vi "Single_Pulse_Debuger.vi"() -> ()   [LabVIEW 2021]
uses:
  Drivers/Arduino_Pulse_Generator/Configurate/Channel_Pulse_Stream.ctl
  Addons/Prepare_Pulse_Sequence/Pulse_Sequence_Global.vi
panel:
  in  "Unit":string(combo)
  in  "Enum":T1(ring)=enum."initialize"
  in  "Arduino VISA":refnum<visa-resource-name>
  out "pulse seq changed (?)":bool=TRUE
  out "Init outp register 2 (8-13)":bool[](array[boolean])
  out "Init outp register 1 (2-7)":bool[](array[boolean])
  out "Pulse sequence":T2[](array[typedef]) {"channel" min=2 max=13 step=1}
  in  "Run sequence":bool
  in  "Close":bool
  in  "Define pulse sequence":bool
  in  "Define initial states":bool
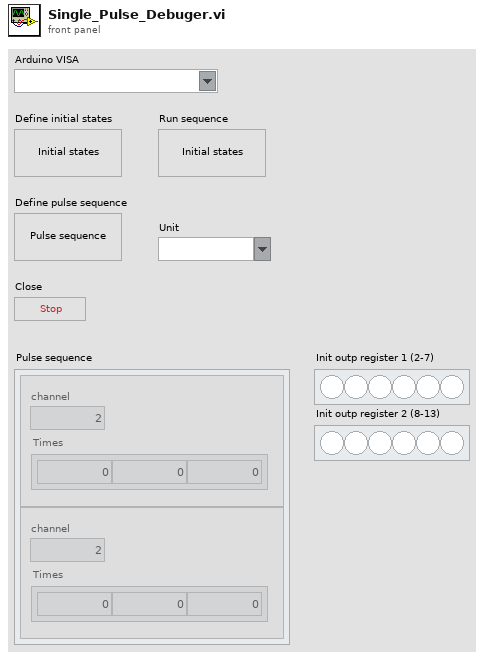
[diagram p1: front panel]
types:
  T1 = enum16{"close", "run", "set pulse", "set initial", "initialize"}
  T2 = typedef "Channel_Pulse_Stream.ctl" = cluster{"Times":dbl[], "channel":u8}
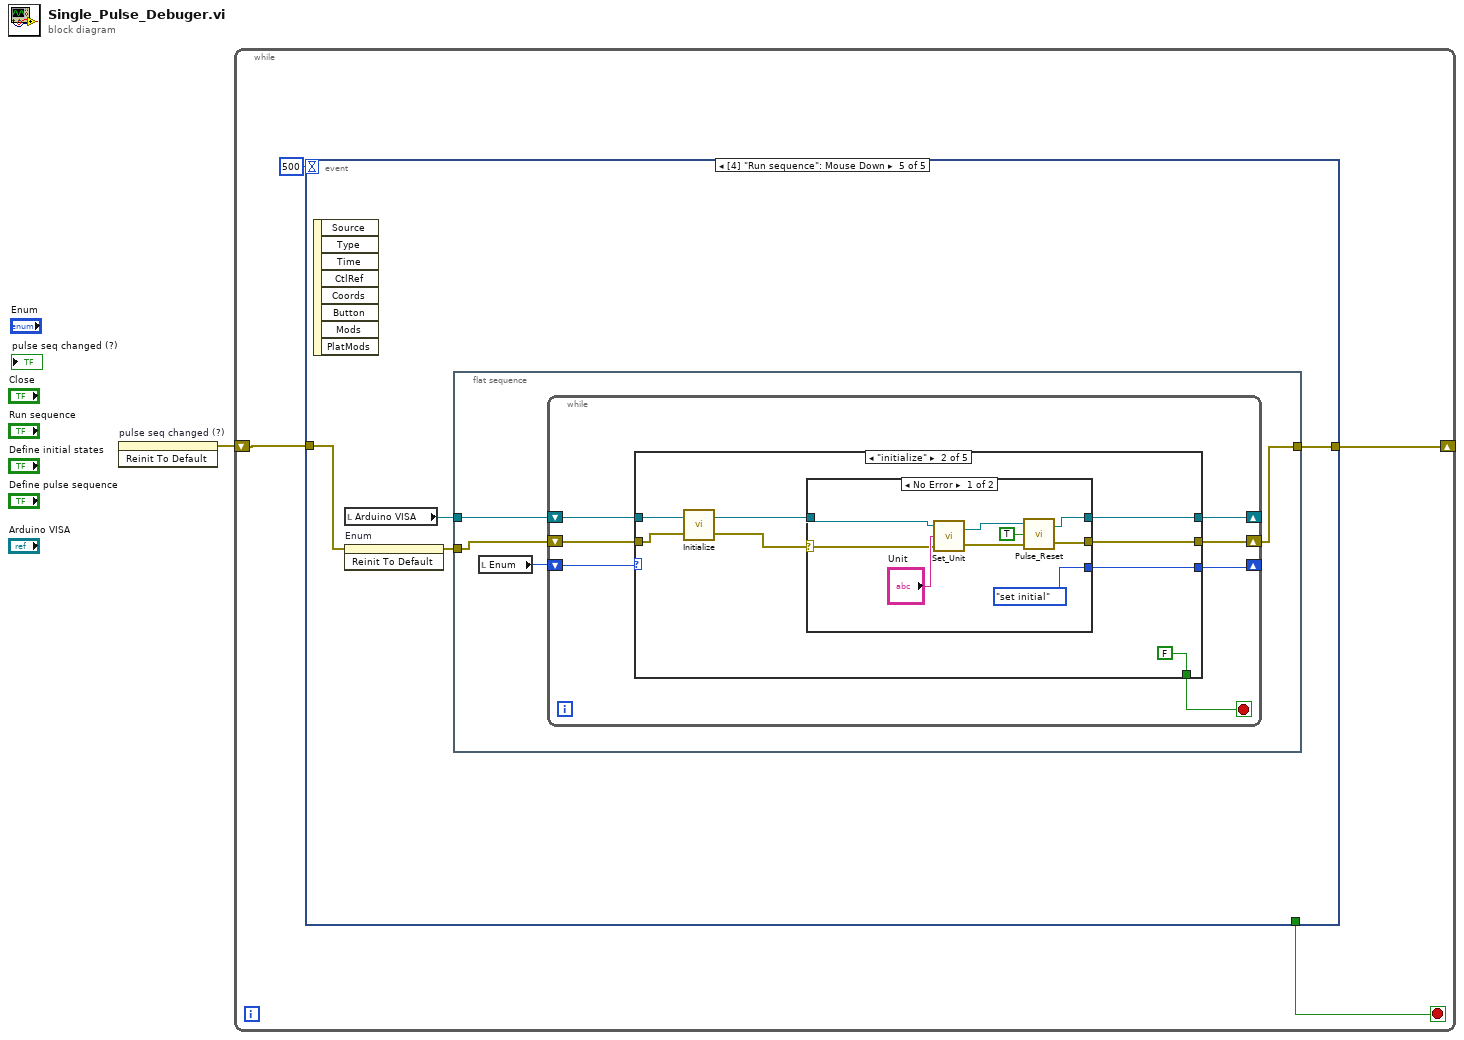
[diagram p0: block diagram]
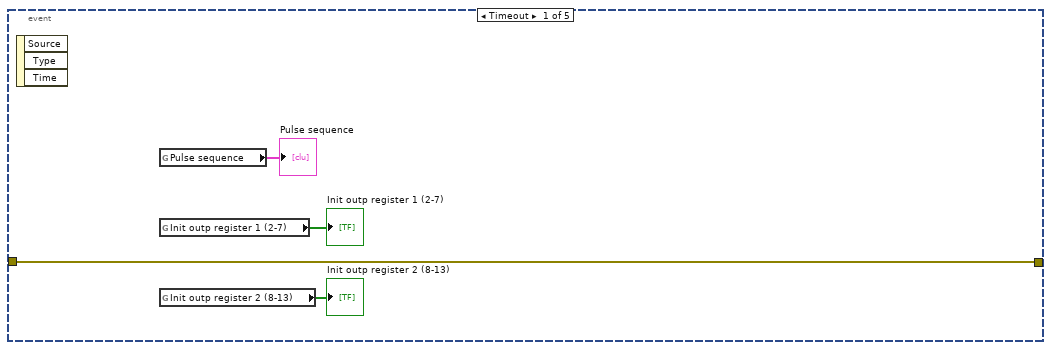
[diagram p2: hidden frame]
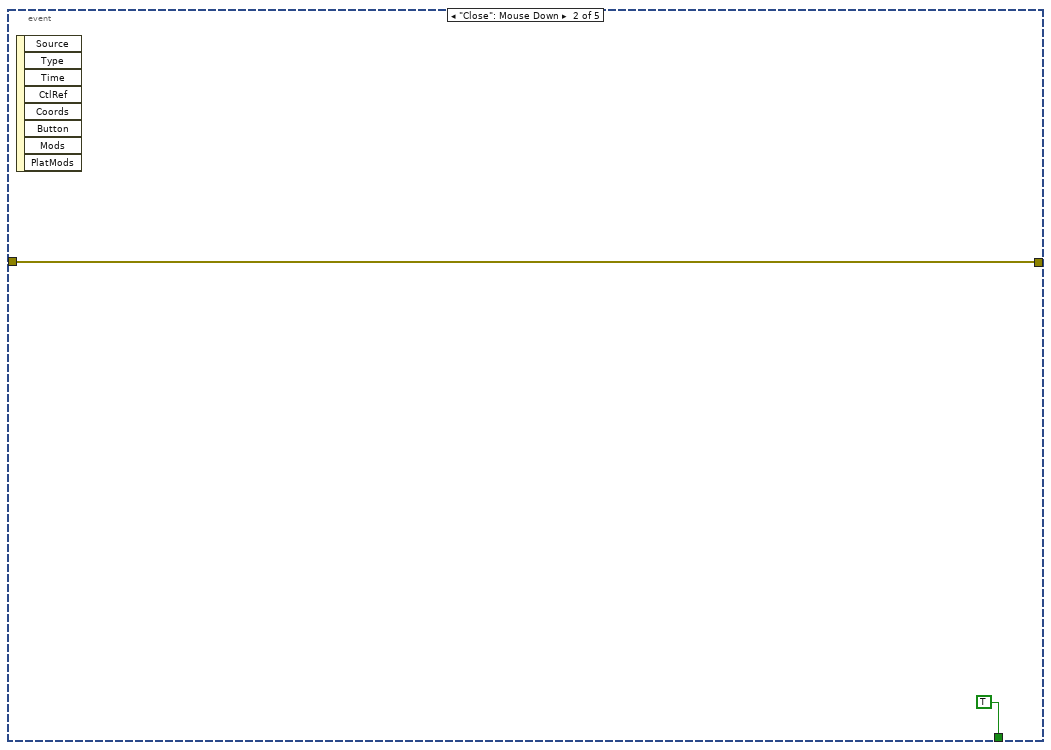
[diagram p3: hidden frame]
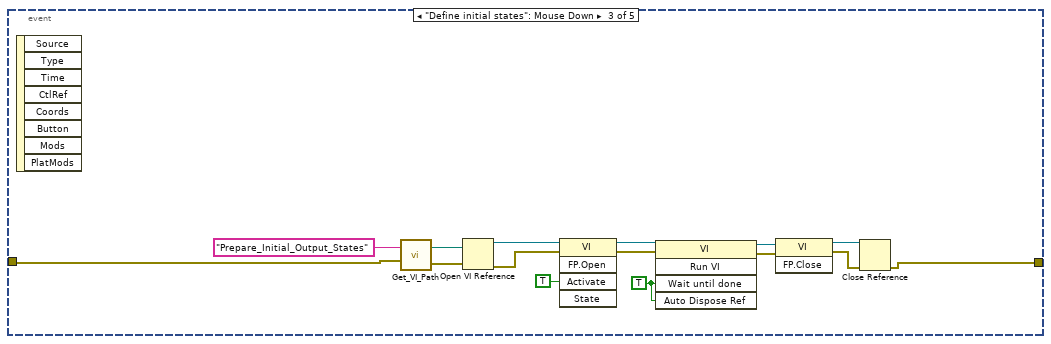
[diagram p4: hidden frame]
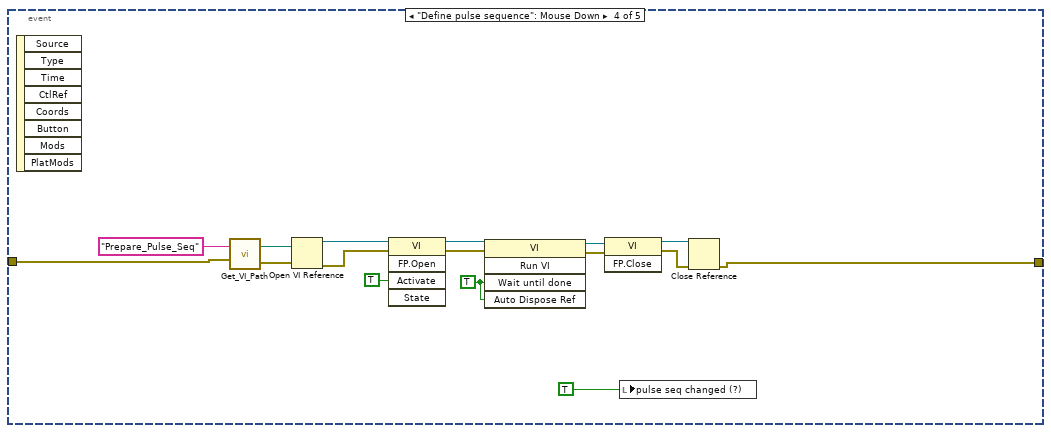
[diagram p5: hidden frame]
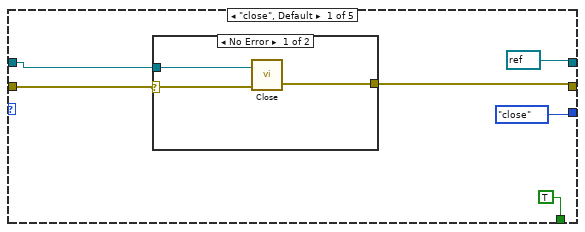
[diagram p6: hidden frame]
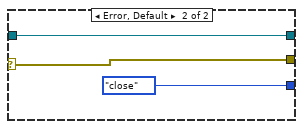
[diagram p8: hidden frame]
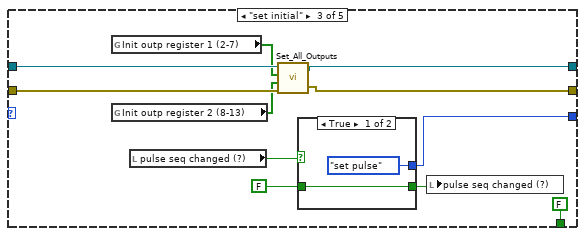
[diagram p9: hidden frame]
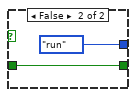
[diagram p10: hidden frame]
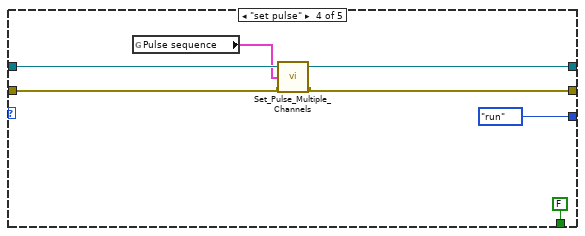
[diagram p11: hidden frame]
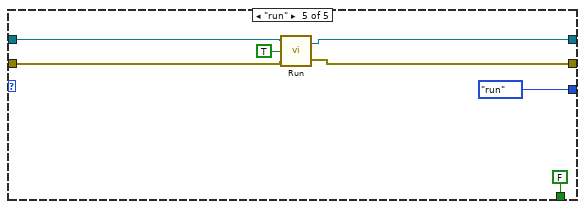
[diagram p12: hidden frame]
diagram:
  n1 = invoke on="pulse seq changed (?)" class="Bool (strict)" method="Reinit To Default"() -> (error out=w1:errorcluster)  [unwired: 3 in, 2 out]
  n2 = while {
    shift-right: [w4] -> _
    shift-left: w1 -> [w5]
    stop <- w2 stop-if-true
    n3 = event shown="[4] \"Run sequence\": Mouse Down" {
      selector: _ -> [_ _ _ _ _]
      dyn-events: _ -> [_ _ _ _ _]
      timeout: 500 -> [_ _ _ _ _]
      tunnel: w5 -> [w6 w10 w13 w29 w44]
      tunnel: [w6 w10 w12 w28 w43] -> w4
      tunnel: [_ TRUE _ _ _] -> w2
      event Timeout {
        n4 = event-data() -> ()  [unwired: 1 in, 3 out]
        n5 = global read "Pulse_Sequence_Global.vi" "Pulse sequence"() -> (→"Pulse sequence":T2[])
        n6 = global read "Pulse_Sequence_Global.vi" "Init outp register 1 (2-7)"() -> (→"Init outp register 1 (2-7)":bool[])
        n7 = global read "Pulse_Sequence_Global.vi" "Init outp register 2 (8-13)"() -> (→"Init outp register 2 (8-13)":bool[])
      }
      event "Close": Mouse Down {
        n8 = event-data() -> ()  [unwired: 1 in, 8 out]
      }
      event "Define initial states": Mouse Down {
        w18 = TRUE ("Wait Until Done")
        n9 = event-data() -> ()  [unwired: 1 in, 8 out]
        n10 = call "Get_VI_Path.vi"("error in"=w13, "VI name (no .vi)"="Prepare_Initial_Output_States") -> ("error out"=w23:errorcluster, "File Path"=w25:path)
        n11 = Open VI Reference(vi path=w25, error in (no error)=w23) -> (vi reference=w24:refnum<vi>, error out=w22:errorcluster)  [unwired: 4 in]
        n12 = invoke class="VI" method="FP.Open"(reference=w24, error in=w22, "Activate"=TRUE ("Activate?")) -> (reference out=w20:refnum<vi>, error out=w19:errorcluster)  [unwired: 2 in, 3 out]
        n13 = invoke class="VI" method="Run VI"(reference=w20, error in=w19, "Wait until done"=w18, "Auto Dispose Ref"=w18) -> (reference out=w17:refnum<vi>, error out=w16:errorcluster)  [unwired: 1 in, 3 out]
        n14 = invoke class="VI" method="FP.Close"(reference=w17, error in=w16) -> (reference out=w15:refnum<vi>, error out=w14:errorcluster)  [unwired: 1 in, 1 out]
        n15 = Close Reference(reference=w15, error in (no error)=w14) -> (error out=w12:errorcluster)
      }
      event "Define pulse sequence": Mouse Down {
        w34 = TRUE ("Wait Until Done")
        n16 = event-data() -> ()  [unwired: 1 in, 8 out]
        n17 = call "Get_VI_Path.vi"("error in"=w29, "VI name (no .vi)"="Prepare_Pulse_Seq") -> ("error out"=w39:errorcluster, "File Path"=w41:path)
        n18 = Open VI Reference(vi path=w41, error in (no error)=w39) -> (vi reference=w40:refnum<vi>, error out=w38:errorcluster)  [unwired: 4 in]
        n19 = invoke class="VI" method="FP.Open"(reference=w40, error in=w38, "Activate"=TRUE ("Activate?")) -> (reference out=w36:refnum<vi>, error out=w35:errorcluster)  [unwired: 2 in, 3 out]
        n20 = invoke class="VI" method="Run VI"(reference=w36, error in=w35, "Wait until done"=w34, "Auto Dispose Ref"=w34) -> (reference out=w33:refnum<vi>, error out=w32:errorcluster)  [unwired: 1 in, 3 out]
        n21 = invoke class="VI" method="FP.Close"(reference=w33, error in=w32) -> (reference out=w31:refnum<vi>, error out=w30:errorcluster)  [unwired: 1 in, 1 out]
        n22 = local write "pulse seq changed (?)"(TRUE ("pulse seq changed (?)")) -> ()
        n23 = Close Reference(reference=w31, error in (no error)=w30) -> (error out=w28:errorcluster)
      }
      event "Run sequence": Mouse Down {
        n24 = event-data() -> ()  [unwired: 1 in, 8 out]
        n25 = local read "Arduino VISA"() -> (w45:refnum<visa-resource-name>)
        n26 = invoke on="Enum" class="Enum (strict)" method="Reinit To Default"(error in=w44) -> (error out=w46:errorcluster)  [unwired: 2 in, 2 out]
        n27 = flat-sequence {
          tunnel: w46 -> [w49]
          tunnel: w45 -> [w50]
          tunnel: [w48] -> w43
          frame #0 {
            n28 = local read "Enum"() -> (w47:T1)
            n29 = while {
              shift-right: [w53] -> _
              shift-left: w47 -> [w51]
              shift-right: [w55] -> _
              shift-left: w50 -> [w57]
              shift-right: [w54] -> w48
              shift-left: w49 -> [w56]
              stop <- w52 stop-if-true
              n30 = case shown="\"initialize\"" w51 {
                tunnel: w57 -> [w63 w75 w97 w105 w115]
                tunnel: w56 -> [w59 w69 w95 w108 w113]
                tunnel: [refnum<visa-resource-name> refnum ("Arduino VISA") w74 w96 w106 w114] -> w55
                tunnel: [w62 w73 w94 w107 w112] -> w54
                tunnel: [T1."close" ("Enum") w72 w98 T1."run" ("Enum") T1."run" ("Enum")] -> w53
                tunnel: [TRUE FALSE FALSE FALSE FALSE] -> w52
                frame "close", Default {
                  n31 = case shown="No Error" w59 {
                    selector: w59 -> [w64 w67]
                    tunnel: w63 -> [w66 _]
                    tunnel: [w65 w67] -> w62
                    frame No Error {
                      n32 = call "Close.vi"("error in"=w64, "VISA arduino in"=w66) -> ("error out"=w65:errorcluster)  [unwired: 1 in]
                    }
                    frame Error {
                    }
                  }
                }
                frame "initialize" {
                  n33 = call "Initialize.vi"("error in"=w69, "VISA arduino in"=w75) -> ("error out"=w68:errorcluster, "VISA arduino out"=w70:refnum<visa-resource-name>)
                  n34 = case shown="No Error" w68 {
                    selector: w68 -> [w76 w86]
                    tunnel: [w79 w85] -> w74
                    tunnel: [w80 w86] -> w73
                    tunnel: [T1."set initial" ("Enum") T1."close" ("Enum")] -> w72
                    tunnel: w70 -> [w77 w85]
                    frame No Error {
                      n35 = call "Set_Unit.vi"("error in"=w76, "Unit"="Unit", "VISA arduino in"=w77) -> ("error out"=w81:errorcluster, "VISA arduino out"=w82:refnum<visa-resource-name>)
                      n36 = call "Pulse_Reset.vi"("error in"=w81, "reset?"=TRUE, "VISA arduino in"=w82) -> ("error out"=w80:errorcluster, "VISA arduino out"=w79:refnum<visa-resource-name>)
                    }
                    frame Error, Default {
                    }
                  }
                }
                frame "set initial" {
                  n37 = global read "Pulse_Sequence_Global.vi" "Init outp register 1 (2-7)"() -> (w93:bool[])
                  n38 = global read "Pulse_Sequence_Global.vi" "Init outp register 2 (8-13)"() -> (w92:bool[])
                  n39 = local read "pulse seq changed (?)"() -> (w91:bool)
                  n40 = call "Set_All_Outputs.vi"("error in"=w95, "register 2 (8-13)"=w92, "register 1 (2-7)"=w93, "VISA arduino in"=w97) -> ("error out"=w94:errorcluster, "VISA arduino out"=w96:refnum<visa-resource-name>)
                  n41 = case shown="True" w91 {
                    tunnel: [T1."set pulse" ("Enum") T1."run" ("Enum")] -> w98
                    tunnel: [w99 w101] -> w90
                    tunnel: FALSE -> [w99 w101]
                    frame True {
                    }
                    frame False {
                    }
                  }
                  n42 = local write "pulse seq changed (?)"(w90) -> ()
                }
                frame "set pulse" {
                  n43 = global read "Pulse_Sequence_Global.vi" "Pulse sequence"() -> (w104:T2[])
                  n44 = call "Set_Pulse_Multiple_Channels.vi"("error in"=w108, "Pulses"=w104, "VISA arduino in"=w105) -> ("error out"=w107:errorcluster, "VISA arduino out"=w106:refnum<visa-resource-name>)  [unwired: 1 in]
                }
                frame "run" {
                  n45 = call "Run.vi"("error in"=w113, "run?"=TRUE, "VISA arduino in"=w115) -> ("error out"=w112:errorcluster, "VISA arduino out"=w114:refnum<visa-resource-name>)
                }
              }
            }
          }
        }
      }
    }
  }
